vi "Read Control Props.vi"(8 "error in (no error)":errorcluster, 11 "ButtonControlEditorPanel in":refnum<class "ButtonControlEditorPanel.lvclass">) -> (0 "error out":errorcluster, 2 "Control Props":T1, 3 "ButtonControlEditorPanel out":refnum<class "ButtonControlEditorPanel.lvclass">)   [LabVIEW 2020, in "VolatusGUIControls.lvlib" / "ButtonControlEditorPanel.lvclass"]
uses:
  ButtonControlEditorPanel.lvclass
  Control Props.ctl
  ButtonControlEditorPanel.lvclass/ButtonControlEditorPanel.ctl
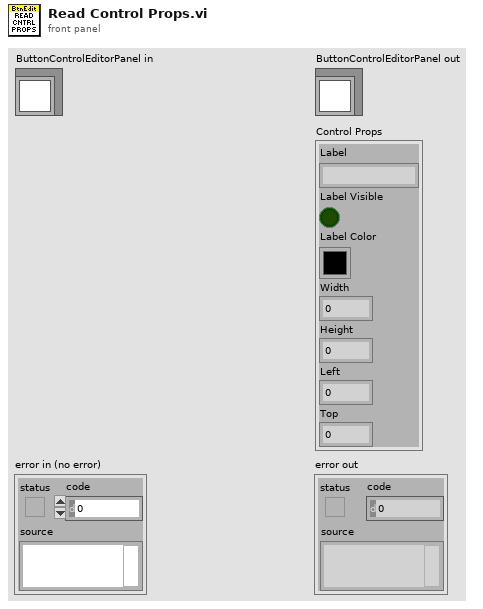
[diagram p1: front panel]
types:
  T1 = typedef "VolatusGUIControls.lvlib/ButtonControlEditorPanel.lvclass/Control Props.ctl" = cluster{"Label":string, "Label Visible":bool, "Label Color":u32, "Width":u16, "Height":u16, "Left":i32, "Top":i32}
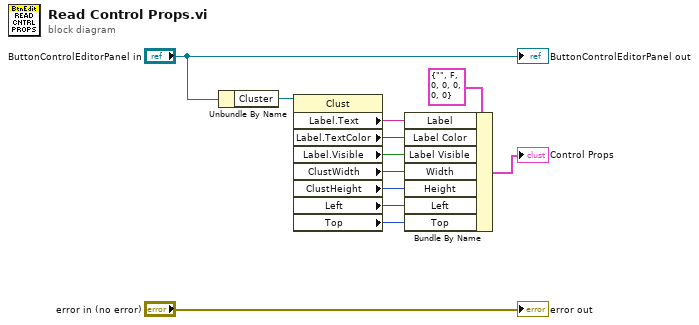
[diagram p0: block diagram]
diagram:
  n1 = Unbundle By Name("ButtonControlEditorPanel in") -> ("Cluster"=w10:refnum<vi>)
  n2 = property class="Clust"(reference=w10) -> ("Label.Text"=w8:string, "Label.TextColor"=w7:u32, "Label.Visible"=w6:bool, "ClustWidth"=w4:u32, "ClustHeight"=w3:u32, "Left"=w2:i32, "Top"=w1:i32)  [unwired: 1 in, 2 out]
  n3 = Bundle By Name(cluster=T1 {"Label"="", "Label Visible"=FALSE, "Label Color"=0, "Width"=0, "Height"=0, "Left"=0, "Top"=0} ("Control Props"), "Label"=w8, "Label Color"=w7, "Label Visible"=w6, "Width"=w4, "Height"=w3, "Left"=w2, "Top"=w1) -> (→"Control Props":T1)
  "error out" <- "error in (no error)"
  "ButtonControlEditorPanel out" <- "ButtonControlEditorPanel in"
